vi "ep_Speed Estimation for SVAF (ICM).vi"(0 "SVAF spectrum":cluster{"f0":dbl, "df":dbl, "spectrum":dbl[]}, 5 "fundamental frequency [Hz]":dbl format="%#_13g", 7 "nominal frequency":enum16{"50 Hz", "60 Hz"}(ring), 9 "nameplate speed":T1, 11 "error in (no error)":errorcluster, 12 "last valid window":i32) -> (3 "candidate speeds":cluster{"speed [RPM]":dbl, "slip":dbl}[](array[cluster]), 4 "speed data":cluster{"speed [RPM]":dbl, "slip":dbl}={"speed [RPM]"=nan, "slip"=nan}, 14 "current valid window":i32, 15 "error out":errorcluster)   [LabVIEW 2017]
uses:
  <vilib>/addons/Electrical Power/Motor Monitoring/NI_EP_Motor Monitoring.lvlib
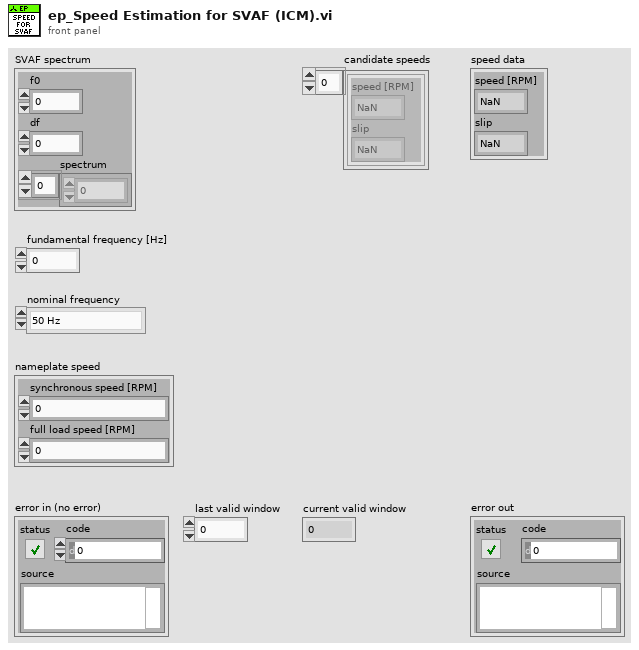
[diagram p1: front panel]
types:
  T1 = cluster{"synchronous speed [RPM]":dbl, "full load speed [RPM]":dbl}
  T2 = cluster{"frequency":dbl[], "magnitude [dB]":dbl[]}
  T3 = cluster{"frequency in window":dbl[], "magnitude in window":dbl[], "enough points for peak search?":bool, "max magnitude in window":dbl}[]
  T4 = cluster{"maximum speed":dbl, "minimum speed":dbl}
  T5 = cluster{"original peak frequency":dbl[], "fitted peak frequency":dbl[], "fitted peak magnitude":dbl[]}[]
  T6 = typedef "NI_EP_Motor Monitoring.lvlib/ep_Harmonic for Speed Calculation.ctl" = enum16{"invalid", "fr", "2fs-2fr", "2fs-fr", "2fr"}
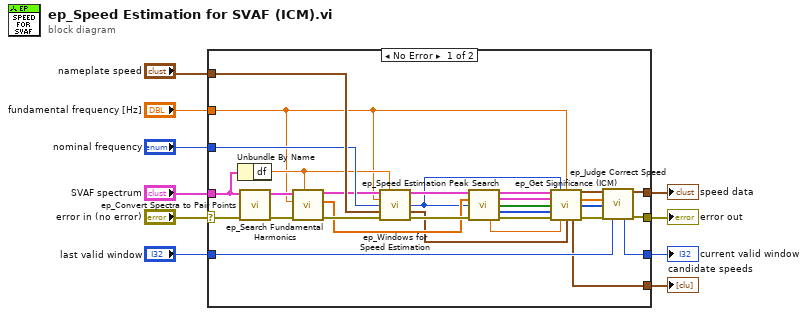
[diagram p0: block diagram]
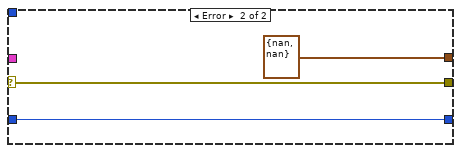
[diagram p2: hidden frame]
diagram:
  n1 = case shown="No Error" "error in (no error)" {
    selector: "error in (no error)" -> [w34 w43]
    tunnel: [w26 w43] -> w9
    tunnel: "fundamental frequency [Hz]" -> [w14 _]
    tunnel: "nameplate speed" -> [w40 _]
    tunnel: "SVAF spectrum" -> [w30 _]
    tunnel: [w25 cluster{"speed [RPM]":dbl, "slip":dbl} {"speed [RPM]"=nan, "slip"=nan} ("speed data")] -> w6
    tunnel: "nominal frequency" -> [w32 _]
    tunnel: "last valid window" -> [w20 w41]
    tunnel: [w19 w41] -> w2
    tunnel: [w11 _] -> w1
    frame No Error {
      n2 = Unbundle By Name(w30) -> ("df"=w18:dbl)
      n3 = call <vilib>:"ep_Convert Spectra to Pair Points.vi"("error in (no error)"=w34, "spectra"=w30) -> ("error out"=w33:errorcluster, "spectra points"=w28:T2)  [unwired: 6 in, 2 out]
      n4 = call <vilib>:"ep_Search Fundamental Harmonics.vi"("df"=w18, "error in (no error)"=w33, "fundamental frequency [Hz]"=w14, "all spectra points"=w28) -> ("error out"=w39:errorcluster, "fundamental harmonics frequencies"=w17:dbl[], "dup all spectra points"=w31:cluster{"frequency":dbl[], "magnitude":dbl[]})  [unwired: 5 in]
      n5 = call <vilib>:"ep_Windows for Speed Estimation.vi"("all spectra points"=w31, "df"=w18, "fundamental frequency [Hz]"=w14, "nominal frequency"=w32, "nameplate speed"=w40, "error in (no error)"=w39) -> ("points in window"=w29:T3, "pole pairs"=w15:i32, "range of speed"=w13:T4, "error out"=w38:errorcluster)  [unwired: 6 in]
      n6 = call <vilib>:"ep_Speed Estimation Peak Search.vi"("spectra points in window"=w29, "frequencies excluded"=w17, "pole pairs"=w15, "error in (no error)"=w38) -> ("dup spectra points in window"=w37:T3, "peaks information"=w36:T5, "enough points for peak search?"=w24:bool[], "number of peaks"=w23:i32[], "minimum max-magnitude"=w12:dbl, "error out"=w35:errorcluster)  [unwired: 6 in]
      n7 = call <vilib>:"ep_Get Significance (ICM).vi"("spectra points in window"=w37, "pole pairs"=w15, "fundamental frequency [Hz]"=w14, "peaks information"=w36, "enough points for peak search?"=w24, "number of peaks"=w23, "error in (no error)"=w35, "minimum max-magnitude"=w12, "range of speed"=w13) -> ("top3 speed data"=w16:cluster{"speed [RPM]":dbl, "slip":dbl}[], "top3 significance"=w22:dbl[], "top3 harmonic for speed calculation"=w21:T6[], "candidate speeds"=w11:cluster{"speed [RPM]":dbl, "slip":dbl}[], "error out"=w27:errorcluster)  [unwired: 2 in]
      n8 = call <vilib>:"ep_Judge Correct Speed.vi"("top3 speed data"=w16, "top3 significance"=w22, "top3 harmonic for speed calculation"=w21, "error in (no error)"=w27, "last valid window"=w20) -> ("speed data"=w25:cluster{"speed [RPM]":dbl, "slip":dbl}, "current valid window"=w19:i32, "error out"=w26:errorcluster)  [unwired: 8 in]
    }
    frame Error {
    }
  }
  "error out" <- w9
  "speed data" <- w6
  "current valid window" <- w2
  "candidate speeds" <- w1
